vi "MakeFailsafeCode.vi"() -> (3 "resulting string":string)   [LabVIEW 2023]
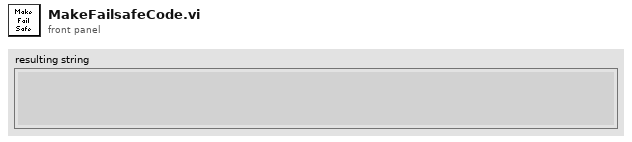
[diagram p1: front panel]
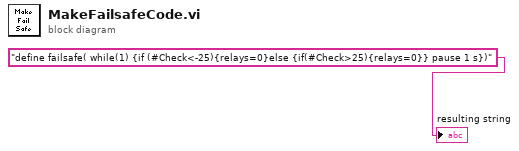
[diagram p0: block diagram]
diagram:
  "resulting string" <- "define failsafe( while(1) {if (#Check<-25){relays=0}else {if(#Check>25){relays=0}} pause 1 s})" ("Command")
